vi "Create RBCIA.vi"(10 "Camera image mapping":T1(array[cluster])=[{"CameraName"="Cam1", "ImageLabel"="C1"}, {"CameraName"="Cam2", "ImageLabel"="C2"}, {"CameraName"="Cam3", "ImageLabel"="C3"}, {"CameraName"="Cam4", "ImageLabel"="C4"}, {"CameraName"="Cam5", "ImageLabel"="C5"}, {"CameraName"="Cam6", "ImageLabel"="C6"}], 11 "Inspection.Image details_init":T2(array[cluster])) -> (3 "RBCIA (Rack based camera image indicator mapping) out":cluster{"Rack Id":u8, "Label names":string[]}[](array[cluster]))   [LabVIEW 2019, in "ZenGage v3.0 UI.lvclass"]
uses:
  ZenGage v3.0 UI.lvclass
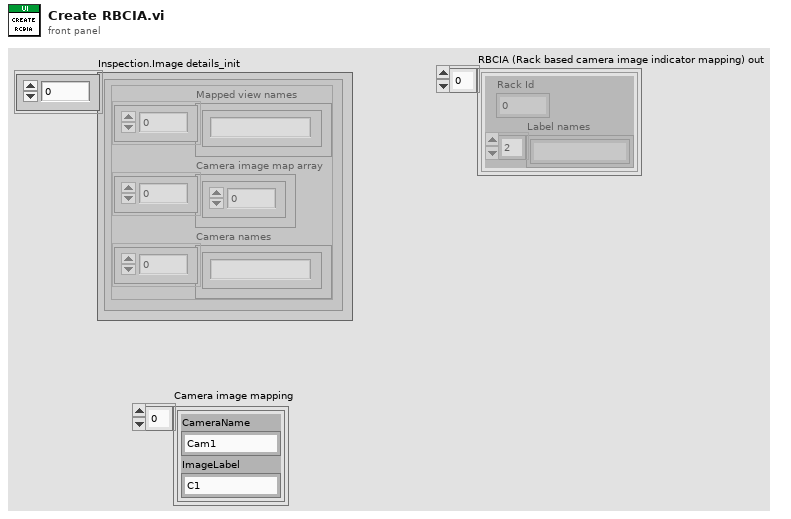
[diagram p1: front panel]
types:
  T1 = cluster{"CameraName":string, "ImageLabel":string}[]
  T2 = cluster{"Mapped view names":string[], "Camera image map array":i32[], "Camera names":string[]}[]
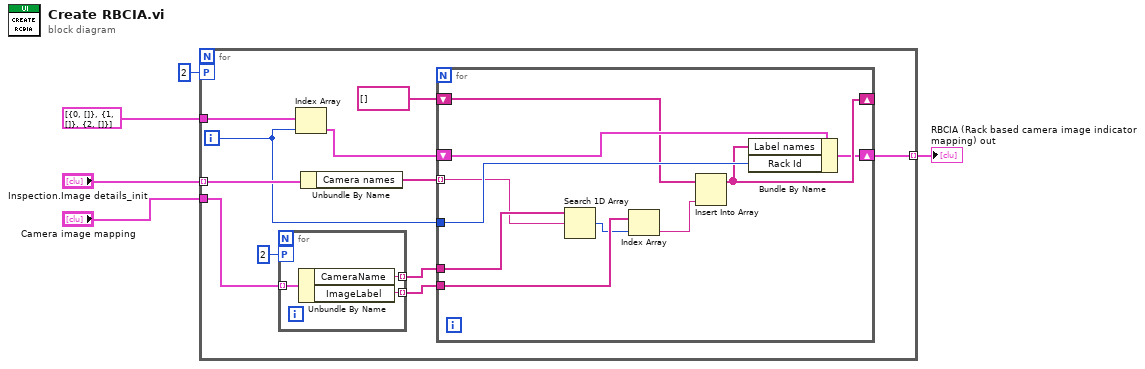
[diagram p0: block diagram]
diagram:
  n1 = for {
    tunnel: "Inspection.Image details_init" -> [w16] mode=indexing
    tunnel: "Camera image mapping" -> [w11]
    tunnel: cluster{"Rack Id":u8, "Label names":string[]}[] [{"Rack Id"=0, "Label names"=[]}, {"Rack Id"=1, "Label names"=[]}, {"Rack Id"=2, "Label names"=[]}] ("RBCIA (Rack based camera image indicator mapping)") -> [w15]
    tunnel: [w7] -> w2 mode=indexing
    workers-P: 2 -> [_]
    i -> [w12]
    n2 = for {
      tunnel: w11 -> [w19] mode=indexing
      tunnel: [w18] -> w10 mode=indexing
      tunnel: [w17] -> w9 mode=indexing
      workers-P: 2 -> [_]
      n3 = Unbundle By Name(w19) -> ("CameraName"=w18:string, "ImageLabel"=w17:string)
    }
    n4 = Index Array(array=w15, index=w12) -> (element=w14:cluster{"Rack Id":u8, "Label names":string[]})
    n5 = Unbundle By Name(w16) -> ("Camera names"=w13:string[])
    n6 = for {
      tunnel: w13 -> [w26] mode=indexing
      tunnel: w12 -> [w28]
      tunnel: w10 -> [w27]
      tunnel: w9 -> [w25]
      shift-right: [w22] -> _
      shift-left: string[] [] -> [w21]
      shift-right: [w20] -> w7
      shift-left: w14 -> [w29]
      n7 = Search 1D Array(1D array=w27, element=w26) -> (index of element=w24:i32)  [unwired: 1 in]
      n8 = Index Array(array=w25, index=w24) -> (element=w23:string)
      n9 = Insert Into Array(array=w21, new element=w23) -> (w22:string[])  [unwired: 1 in]
      n10 = Bundle By Name(cluster=w29, "Label names"=w22, "Rack Id"=w28) -> (w20:cluster{"Rack Id":u8, "Label names":string[]})
    }
  }
  "RBCIA (Rack based camera image indicator mapping) out" <- w2
